vi "ptr_read.vi"() -> ()   [LabVIEW 2013]
panel:
  in  "ptr_read":i32
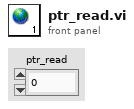
[diagram p1: front panel]
diagram:
